vi "LM_II_11_15 - Copy.vi"   [LabVIEW 2012]
uses:
  <vilib>/NXT/Subs/MotorOutput.ctl
  <vilib>/NXT/Block Support/NXT_InputPort.ctl
  <vilib>/NXT/Block Support/NXT_MessageMailbox.ctl
  <vilib>/NXT/Block Support/NXT_OutputPort.ctl
  <vilib>/NXT/Block Support/NXT_TimerIndex.ctl
types:
  T1 = typedef "MotorOutput.ctl" = u8
  T2 = typedef "LVHSConnector.ctl" = refnum<class "BrickReference.lvclass">
  T3 = typedef "NXT_InputPort.ctl" = u32
  T4 = typedef "NXT_MessageMailbox.ctl" = u8
  T5 = typedef "NXT_OutputPort.ctl" = u8
  T6 = typedef "NXT_TimerIndex.ctl" = u8
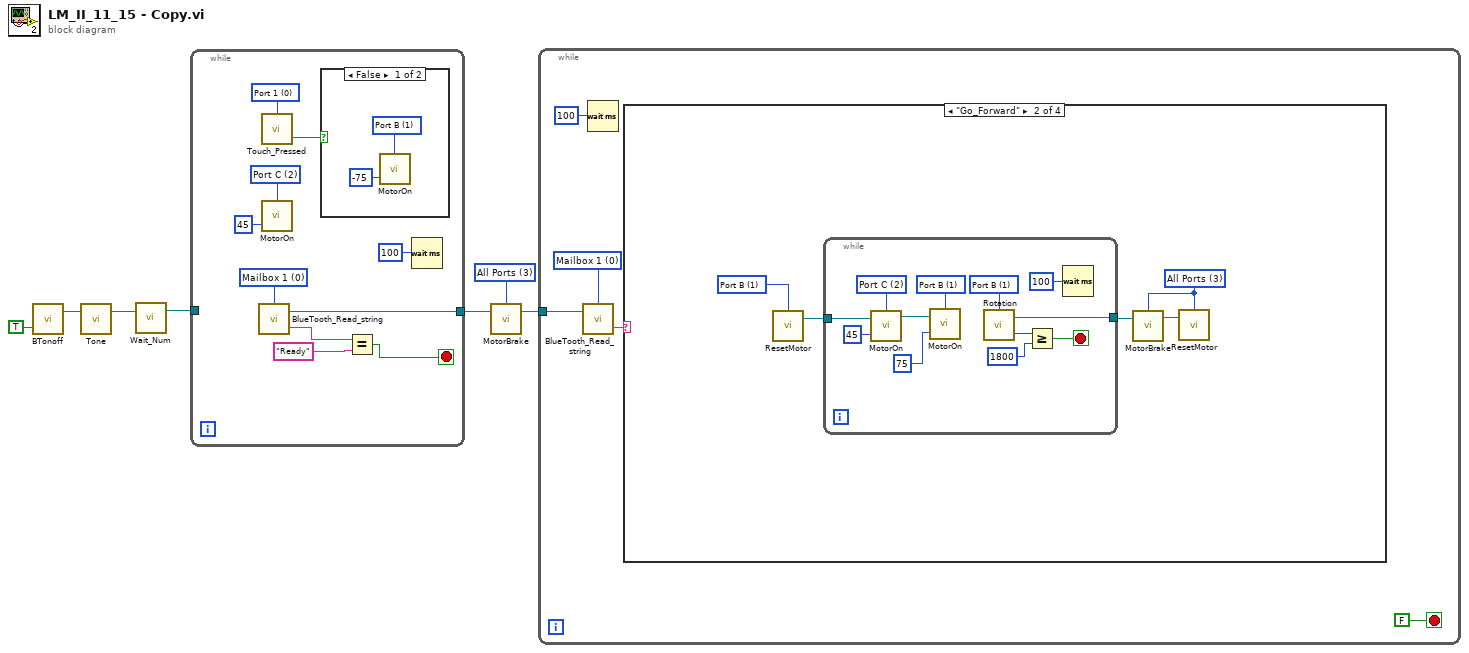
[diagram p0: block diagram]
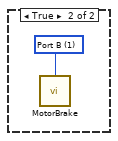
[diagram p2: hidden frame]
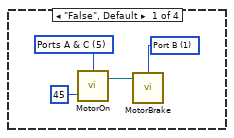
[diagram p3: hidden frame]
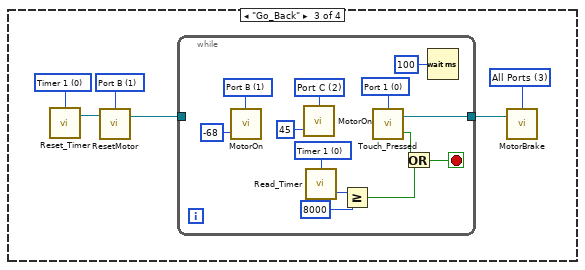
[diagram p4: hidden frame]
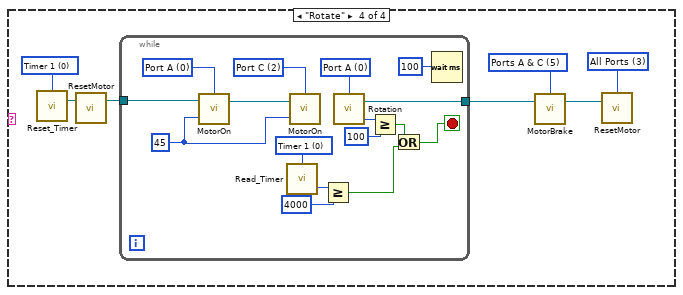
[diagram p5: hidden frame]
diagram:
  w2 = T1 3 items=["Port A"=0, "Port B"=1, "Port C"=2, "Ports A & B"=4, "Ports A & C"=5, "Ports B & C"=6, "All Ports"=3] ("Port (All Ports)")
  n1 = call <vilib>:"BTonoff.vi"("On/Off"=TRUE) -> ("NXT/EV3"=w6:T2)  [unwired: 2 in, 1 out]
  n2 = call <vilib>:"Tone.vi"("NXT/EV3"=w6) -> ("NXT/EV3"=w5:T2)  [unwired: 3 in]
  n3 = call <vilib>:"Wait_Num.vi"("NXT/EV3"=w5) -> ("NXT/EV3"=w4:T2)  [unwired: 3 in]
  n4 = while {
    tunnel: w4 -> [_]
    tunnel: [w9] -> w1
    stop <- w8 stop-if-true
    w12 = T1 2 items=["Port A"=0, "Port B"=1, "Port C"=2, "Ports A & B"=4, "Ports A & C"=5, "Ports B & C"=6, "All Ports"=3] ("Output Port (All Ports)")
    w14 = T3 0 items=["Port 1", "Port 2", "Port 3", "Port 4"] ("Port (Port 1)")
    w17 = T4 0 items=["Mailbox 1", "Mailbox 2", "Mailbox 3", "Mailbox 4", "Mailbox 5", "Mailbox 6", "Mailbox 7", "Mailbox 8", "Mailbox 9", "Mailbox 10"] ("Mailbox")
    n5 = call <vilib>:"BlueTooth_Read_string.vi"("Mailbox"=w17) -> ("Message"=w16:string, "NXT/EV3"=w9:T2)  [unwired: 2 in]
    n6 = call <vilib>:"Touch_Pressed.vi"("Port (Port 1)"=w14) -> ("Yes / No"=w13:bool)  [unwired: 2 in, 1 out]
    n7 = call <vilib>:"MotorOn.vi"("Power (75)"=45, "Output Port (All Ports)"=w12) -> ()  [unwired: 2 in, 1 out]
    n8 = case shown="False" w13 {
      frame False {
        w19 = T1 1 items=["Port A"=0, "Port B"=1, "Port C"=2, "Ports A & B"=4, "Ports A & C"=5, "Ports B & C"=6, "All Ports"=3] ("Output Port (All Ports)")
        n9 = call <vilib>:"MotorOn.vi"("Power (75)"=-75, "Output Port (All Ports)"=w19) -> ()  [unwired: 2 in, 1 out]
      }
      frame True {
        w20 = T1 1 items=["Port A"=0, "Port B"=1, "Port C"=2, "Ports A & B"=4, "Ports A & C"=5, "Ports B & C"=6, "All Ports"=3] ("Port (All Ports)")
        n10 = call <vilib>:"MotorBrake.vi"("Port (All Ports)"=w20) -> ()  [unwired: 3 in, 1 out]
      }
    }
    n11 = Equal?(x=w16, y="Ready") -> (x = y?=w8:bool)
    n12 = Wait (ms)(milliseconds to wait=u32 100) -> ()  [unwired: 1 out]
  }
  n13 = call <vilib>:"MotorBrake.vi"("NXT/EV3"=w1, "Port (All Ports)"=w2) -> ("NXT/EV3"=w3:T2)  [unwired: 2 in]
  n14 = while {
    tunnel: w3 -> [w21]
    stop <- FALSE stop-if-true
    w23 = T4 0 items=["Mailbox 1", "Mailbox 2", "Mailbox 3", "Mailbox 4", "Mailbox 5", "Mailbox 6", "Mailbox 7", "Mailbox 8", "Mailbox 9", "Mailbox 10"] ("Mailbox")
    n15 = call <vilib>:"BlueTooth_Read_string.vi"("NXT/EV3"=w21, "Mailbox"=w23) -> ("Message"=w24:string)  [unwired: 1 in, 1 out]
    n16 = Wait (ms)(milliseconds to wait=u32 100) -> ()  [unwired: 1 out]
    n17 = case shown="\"Go_Forward\"" w24 {
      frame "False", Default {
        w26 = T1 1 items=["Port A"=0, "Port B"=1, "Port C"=2, "Ports A & B"=4, "Ports A & C"=5, "Ports B & C"=6, "All Ports"=3] ("Port (All Ports)")
        w29 = T1 5 items=["Port A"=0, "Port B"=1, "Port C"=2, "Ports A & B"=4, "Ports A & C"=5, "Ports B & C"=6, "All Ports"=3] ("Output Port (All Ports)")
        n18 = call <vilib>:"MotorOn.vi"("Power (75)"=45, "Output Port (All Ports)"=w29) -> ("NXT/EV3"=w27:T2)  [unwired: 2 in]
        n19 = call <vilib>:"MotorBrake.vi"("NXT/EV3"=w27, "Port (All Ports)"=w26) -> ()  [unwired: 2 in, 1 out]
      }
      frame "Go_Forward" {
        w30 = T1 3 items=["Port A"=0, "Port B"=1, "Port C"=2, "Ports A & B"=4, "Ports A & C"=5, "Ports B & C"=6, "All Ports"=3] ("Port (All Ports)")
        w34 = T1 1 items=["Port A"=0, "Port B"=1, "Port C"=2, "Ports A & B"=4, "Ports A & C"=5, "Ports B & C"=6, "All Ports"=3] ("Port (All Ports)")
        n20 = call <vilib>:"ResetMotor.vi"("Port (All Ports)"=w34) -> ("NXT/EV3"=w33:T2)  [unwired: 3 in]
        n21 = while {
          tunnel: w33 -> [w45]
          tunnel: [w41] -> w31
          stop <- w43 stop-if-true
          w37 = T1 1 items=["Port A"=0, "Port B"=1, "Port C"=2, "Ports A & B"=4, "Ports A & C"=5, "Ports B & C"=6, "All Ports"=3] ("Output Port (All Ports)")
          w44 = T5 1 items=["Port A", "Port B", "Port C", "Port D"] ("Port (Port A)")
          w46 = T1 2 items=["Port A"=0, "Port B"=1, "Port C"=2, "Ports A & B"=4, "Ports A & C"=5, "Ports B & C"=6, "All Ports"=3] ("Output Port (All Ports)")
          n22 = call <vilib>:"MotorOn.vi"("Power (75)"=45, "NXT/EV3"=w45, "Output Port (All Ports)"=w46) -> ("NXT/EV3"=w38:T2)  [unwired: 1 in]
          n23 = call <vilib>:"MotorOn.vi"("Power (75)"=75, "NXT/EV3"=w38, "Output Port (All Ports)"=w37) -> ()  [unwired: 1 in, 1 out]
          n24 = call <vilib>:"Rotation.vi"("Port (Port A)"=w44) -> ("Angle of Rotation"=w35:i32, "NXT/EV3"=w41:T2)  [unwired: 2 in]
          n25 = Greater Or Equal?(x=w35, y=1800) -> (x >= y?=w43:bool)
          n26 = Wait (ms)(milliseconds to wait=u32 100) -> ()  [unwired: 1 out]
        }
        n27 = call <vilib>:"MotorBrake.vi"("NXT/EV3"=w31, "Port (All Ports)"=w30) -> ("NXT/EV3"=w32:T2)  [unwired: 2 in]
        n28 = call <vilib>:"ResetMotor.vi"("NXT/EV3"=w32, "Port (All Ports)"=w30) -> ()  [unwired: 2 in, 1 out]
      }
      frame "Go_Back" {
        w47 = T6 0 items=["Timer 1", "Timer 2", "Timer 3"] ("Timer (Timer 1)")
        w52 = T1 3 items=["Port A"=0, "Port B"=1, "Port C"=2, "Ports A & B"=4, "Ports A & C"=5, "Ports B & C"=6, "All Ports"=3] ("Port (All Ports)")
        w50 = T1 1 items=["Port A"=0, "Port B"=1, "Port C"=2, "Ports A & B"=4, "Ports A & C"=5, "Ports B & C"=6, "All Ports"=3] ("Port (All Ports)")
        n29 = call <vilib>:"Reset_Timer.vi"("Timer (Timer 1)"=w47) -> ("NXT/EV3"=w48:T2)  [unwired: 3 in]
        n30 = call <vilib>:"ResetMotor.vi"("NXT/EV3"=w48, "Port (All Ports)"=w50) -> ("NXT/EV3"=w51:T2)  [unwired: 2 in]
        n31 = while {
          tunnel: w51 -> [_]
          tunnel: [w59] -> w49
          stop <- w57 stop-if-true
          w53 = T6 0 items=["Timer 1", "Timer 2", "Timer 3"] ("Timer (Timer 1)")
          w60 = T3 0 items=["Port 1", "Port 2", "Port 3", "Port 4"] ("Port (Port 1)")
          w63 = T1 2 items=["Port A"=0, "Port B"=1, "Port C"=2, "Ports A & B"=4, "Ports A & C"=5, "Ports B & C"=6, "All Ports"=3] ("Output Port (All Ports)")
          w64 = T1 1 items=["Port A"=0, "Port B"=1, "Port C"=2, "Ports A & B"=4, "Ports A & C"=5, "Ports B & C"=6, "All Ports"=3] ("Output Port (All Ports)")
          n32 = call <vilib>:"MotorOn.vi"("Power (75)"=-68, "Output Port (All Ports)"=w64) -> ()  [unwired: 2 in, 1 out]
          n33 = call <vilib>:"MotorOn.vi"("Power (75)"=45, "Output Port (All Ports)"=w63) -> ()  [unwired: 2 in, 1 out]
          n34 = call <vilib>:"Read_Timer.vi"("Timer (Timer 1)"=w53) -> ("Value (msec)"=w56:u32)  [unwired: 2 in, 1 out]
          n35 = Greater Or Equal?(x=w56, y=u32 8000) -> (x >= y?=w54:bool)
          n36 = call <vilib>:"Touch_Pressed.vi"("Port (Port 1)"=w60) -> ("Yes / No"=w58:bool, "NXT/EV3"=w59:T2)  [unwired: 2 in]
          n37 = Or(x=w58, y=w54) -> (x .or. y?=w57:bool)
          n38 = Wait (ms)(milliseconds to wait=u32 100) -> ()  [unwired: 1 out]
        }
        n39 = call <vilib>:"MotorBrake.vi"("NXT/EV3"=w49, "Port (All Ports)"=w52) -> ()  [unwired: 2 in, 1 out]
      }
      frame "Rotate" {
        w67 = T6 0 items=["Timer 1", "Timer 2", "Timer 3"] ("Timer (Timer 1)")
        w69 = T1 3 items=["Port A"=0, "Port B"=1, "Port C"=2, "Ports A & B"=4, "Ports A & C"=5, "Ports B & C"=6, "All Ports"=3] ("Port (All Ports)")
        w71 = T1 5 items=["Port A"=0, "Port B"=1, "Port C"=2, "Ports A & B"=4, "Ports A & C"=5, "Ports B & C"=6, "All Ports"=3] ("Port (All Ports)")
        n40 = call <vilib>:"Reset_Timer.vi"("Timer (Timer 1)"=w67) -> ("NXT/EV3"=w66:T2)  [unwired: 3 in]
        n41 = call <vilib>:"ResetMotor.vi"("NXT/EV3"=w66) -> ("NXT/EV3"=w72:T2)  [unwired: 3 in]
        n42 = while {
          tunnel: w72 -> [w84]
          tunnel: [w79] -> w70
          stop <- w75 stop-if-true
          w76 = T6 0 items=["Timer 1", "Timer 2", "Timer 3"] ("Timer (Timer 1)")
          w81 = T5 0 items=["Port A", "Port B", "Port C", "Port D"] ("Port (Port A)")
          w85 = 45 ("Power (75)")
          w87 = T1 2 items=["Port A"=0, "Port B"=1, "Port C"=2, "Ports A & B"=4, "Ports A & C"=5, "Ports B & C"=6, "All Ports"=3] ("Output Port (All Ports)")
          w88 = T1 0 items=["Port A"=0, "Port B"=1, "Port C"=2, "Ports A & B"=4, "Ports A & C"=5, "Ports B & C"=6, "All Ports"=3] ("Output Port (All Ports)")
          n43 = call <vilib>:"MotorOn.vi"("Power (75)"=w85, "NXT/EV3"=w84, "Output Port (All Ports)"=w88) -> ("NXT/EV3"=w86:T2)  [unwired: 1 in]
          n44 = call <vilib>:"Read_Timer.vi"("Timer (Timer 1)"=w76) -> ("Value (msec)"=w78:u32)  [unwired: 2 in, 1 out]
          n45 = call <vilib>:"MotorOn.vi"("Power (75)"=w85, "NXT/EV3"=w86, "Output Port (All Ports)"=w87) -> ()  [unwired: 1 in, 1 out]
          n46 = Greater Or Equal?(x=w78, y=u32 4000) -> (x >= y?=w73:bool)
          n47 = call <vilib>:"Rotation.vi"("Port (Port A)"=w81) -> ("Angle of Rotation"=w83:i32, "NXT/EV3"=w79:T2)  [unwired: 2 in]
          n48 = Greater Or Equal?(x=w83, y=100) -> (x >= y?=w74:bool)
          n49 = Or(x=w74, y=w73) -> (x .or. y?=w75:bool)
          n50 = Wait (ms)(milliseconds to wait=u32 100) -> ()  [unwired: 1 out]
        }
        n51 = call <vilib>:"MotorBrake.vi"("NXT/EV3"=w70, "Port (All Ports)"=w71) -> ("NXT/EV3"=w68:T2)  [unwired: 2 in]
        n52 = call <vilib>:"ResetMotor.vi"("NXT/EV3"=w68, "Port (All Ports)"=w69) -> ()  [unwired: 2 in, 1 out]
      }
    }
  }
